vi "Voltage Ratio Input and Digital Output.vi"() -> ()   [LabVIEW 2012, in "Phidget Common.lvlib"]
uses:
  <instrlib>/Phidgets/Phidget Common/Phidget Common.lvlib
  <instrlib>/Phidgets/Phidget Digital Output/Public/DigitalOutputStart.vi
  <instrlib>/Phidgets/Phidget Voltage Ratio Input/Public/VoltageRatioInputStart.vi
  <instrlib>/Phidgets/Phidget Voltage Ratio Input/Public/VoltageRatioInputClose.vi
  <instrlib>/Phidgets/Phidget Digital Output/Public/DigitalOutputClose.vi
  <instrlib>/Phidgets/Phidget Voltage Ratio Input/Phidget Voltage Ratio Input.lvlib
  <instrlib>/Phidgets/Phidget Digital Output/Phidget Digital Output.lvlib
panel:
  in  "Voltage Ratio Input Info":T1={"Serial Number"=-1, "Channel"=0, "Port"=0}
  in  "Digital Output Info":T1={"Serial Number"=-1, "Channel"=0, "Port"=0}
  in  "stop":bool
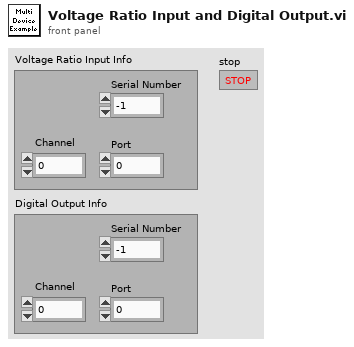
[diagram p1: front panel]
types:
  T1 = cluster{"Serial Number":i32, "Channel":i32, "Port":i32}
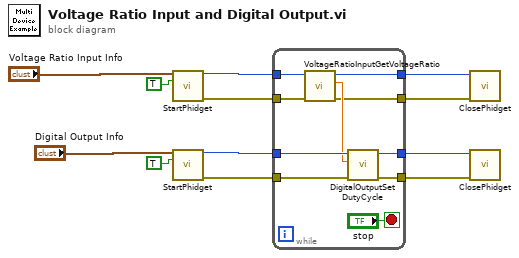
[diagram p0: block diagram]
diagram:
  n1 = call-poly <instrlib>:"StartPhidget.vi"("Device Info"="Voltage Ratio Input Info", "IsHubPort"=TRUE) -> ("Phidget ID"=w12:u64, "error out"=w1:errorcluster)  [unwired: 10 in, 2 out]
  n2 = call-poly <instrlib>:"StartPhidget.vi"("Device Info"="Digital Output Info", "IsHubPort"=TRUE) -> ("Phidget ID"=w11:u64, "error out"=w4:errorcluster)  [unwired: 10 in, 2 out]
  n3 = while {
    tunnel: w1 -> [w22]
    tunnel: w12 -> [w21]
    tunnel: w11 -> [w20]
    tunnel: w4 -> [w19]
    tunnel: [w16] -> w10
    tunnel: [w15] -> w9
    tunnel: [w14] -> w8
    tunnel: [w13] -> w7
    stop <- "stop" stop-if-true
    n4 = call <instrlib>:"VoltageRatioInputGetVoltageRatio.vi"("error in (no error)"=w22, "Device In"=w21) -> ("error out"=w14:errorcluster, "Voltage Ratio"=w18:dbl, "Device Out"=w13:u64)  [unwired: 6 in]
    n5 = call <instrlib>:"DigitalOutputSetDutyCycle.vi"("error in (no error)"=w19, "Duty Cycle"=w18, "Device In"=w20) -> ("error out"=w16:errorcluster, "Device Out"=w15:u64)  [unwired: 6 in]
  }
  n6 = call-poly <instrlib>:"ClosePhidget.vi"("error in"=w8, "Device In"=w7) -> ()  [unwired: 9 in, 1 out]
  n7 = call-poly <instrlib>:"ClosePhidget.vi"("error in"=w10, "Device In"=w9) -> ()  [unwired: 9 in, 1 out]
